vi "HFRR ADV v10.vi"() -> ()   [LabVIEW 2025] (continued)
            n3141 = local read "S 38"() -> (w4253:string)
            n3142 = local read "Temperature before test 2"() -> (w4284:dbl)
            n3143 = local read "Temperature after test 2"() -> (w4274:dbl)
            n3144 = local read "Humidity before test 2"() -> (w4299:dbl)
            n3145 = local read "Humidity after test 2"() -> (w4283:dbl)
            n3146 = local read "MWSD 2"() -> (w4288:dbl)
            n3147 = local read "WS1.4 2"() -> (w4266:dbl)
            n3148 = Concatenate Strings("2)" ("string"), w4248) -> (w4249:string)
            n3149 = Concatenate Strings("3)" ("string"), w4246) -> (w4247:string)
            n3150 = Concatenate Strings("1)" ("string"), w4253) -> (w4252:string)
            n3151 = Concatenate Strings("4)" ("string"), w4243) -> (w4244:string)
            n3152 = Concatenate Strings("5)" ("string"), w4241) -> (w4240:string)
            n3153 = Concatenate Strings("6)" ("string"), w4238) -> (w4237:string)
            n3154 = Concatenate Strings("7)" ("string"), w4234) -> (w4235:string)
            n3155 = Concatenate Strings("8)" ("string"), w4231) -> (w4232:string)
            n3156 = local read "HCF 2"() -> (w4270:dbl)
            n3157 = local read "AVP 2"() -> (w4287:dbl)
            n3158 = local read "s.NO"() -> (w4229:string)
            n3159 = call <vilib>:"New Report.vi"("report type"=enum16{"Standard Report", "HTML"}."Standard Report") -> ("report out"=w4308:refnum<class "NI_report.lvclass">, "error out"=w4307:errorcluster)  [unwired: 13 in]
            n3160 = local read "TITTLE"() -> (w4260:string)
            n3161 = Concatenate Strings(w4285, w4228, w4229, w4285, w4263, w4258, w4285, w4262, w4259, w4285, w4264, w4261, w4285) -> (w4278:string)
            "test by" <- w4278
            n3162 = Number To Fractional String(number=w4284, width (-)=i16 6, precision (6)=i16 2) -> (F-format string=w4273:string)  [unwired: 1 in]
            n3163 = Number To Fractional String(number=w4283, width (-)=i16 6, precision (6)=i16 2) -> (F-format string=w4286:string)  [unwired: 1 in]
            n3164 = Number To Fractional String(number=w4299, width (-)=i16 6, precision (6)=i16 2) -> (F-format string=w4304:string)  [unwired: 1 in]
            n3165 = Number To Fractional String(number=w4288, width (-)=i16 6, precision (6)=i16 2) -> (F-format string=w4290:string)  [unwired: 1 in]
            n3166 = Number To Fractional String(number=w4274, width (-)=i16 6, precision (6)=i16 2) -> (F-format string=w4275:string)  [unwired: 1 in]
            n3167 = Number To Fractional String(number=w4287, width (-)=i16 6, precision (6)=i16 2) -> (F-format string=w4289:string)  [unwired: 1 in]
            n3168 = Number To Fractional String(number=w4270, width (-)=i16 6, precision (6)=i16 2) -> (F-format string=w4269:string)  [unwired: 1 in]
            n3169 = Number To Fractional String(number=w4266, precision (6)=i16 2) -> (F-format string=w4265:string)  [unwired: 2 in]
            n3170 = call-dynamic "Set Report Header Text.vi"("report in"=w4308, "center header text"=w4260, "error in (no error)"=w4307) -> ("report out"=w4279:refnum<class "NI_report.lvclass">, "error out"=w4280:errorcluster)  [unwired: 11 in]
            n3171 = Concatenate Strings(w4268, w4252, w4304, w4268, w4249, w4273, w4268, w4247, w4286, w4268, w4244, w4275, w4268, w4240, w4290, w4268, w4237, w4289, w4268, w4235, w4269, w4268, w4232, w4265) -> (w4256:string)
            "export 2" <- w4256
            n3172 = call-poly <vilib>:"Append Report Text.vi"("report in"=w4279, "text"=w4278, "error in (no error)"=w4280) -> ("report out"=w4282:refnum<class "NI_report.lvclass">, "error out"=w4281:errorcluster)  [unwired: 9 in, 2 out]
            n3173 = local read "test by"() -> (w4255:string)
            n3174 = local read "TITTLE"() -> (w4257:string)
            n3175 = call-poly <vilib>:"Append Report Text.vi"("report in"=w4282, "error in (no error)"=w4281) -> ("report out"=w4303:refnum<class "NI_report.lvclass">, "error out"=w4301:errorcluster)  [unwired: 10 in, 2 out]
            n3176 = Concatenate Strings(w4257, w4256, w4255) -> (→"output":string)
            n3177 = call-poly <vilib>:"Append Report Text.vi"("report in"=w4303, "text"=w4256, "error in (no error)"=w4301) -> ("report out"=w4302:refnum<class "NI_report.lvclass">, "error out"=w4300:errorcluster)  [unwired: 9 in, 2 out]
            n3178 = call-dynamic "Print Report.vi"("report in"=w4302, "printer name (default)"=w4310, "error in (no error)"=w4300) -> ("report out"=w4312:refnum<class "NI_report.lvclass">, "error out"=w4313:errorcluster)  [unwired: 11 in]
            n3179 = call-dynamic "Dispose Report.vi"("report in"=w4312, "error in (no error)"=w4313) -> ()  [unwired: 13 in, 1 out]
          }
        }
        n3180 = case shown="True" "Print 2" {
          frame False {
          }
          frame True {
            n3181 = flat-sequence {
              frame #0 {
                n3182 = local read "s.NO"() -> (→"s.NO 2":string)
                n3183 = Wait (ms)(milliseconds to wait=u32 20) -> ()  [unwired: 1 out]
                n3184 = local read "Sample ID  3"() -> (→"Sample ID  6":string)
                n3185 = local read "Sample ID  4"() -> (→"Sample ID  7":string)
                n3186 = local read "Sample ID"() -> (→"Sample ID  2":string)
                n3187 = local read "Tested by"() -> (→"Tested by 2":string)
                n3188 = local read "Test Date"() -> (→"Test Date 2":string)
                n3189 = local read "Humidity after test 3"() -> (→"Humidity after test 4":dbl)
                n3190 = local read "Ref A Test Date :"() -> (→"TITTLE 4":string)
                n3191 = local read "Temperature before test 3"() -> (w4135:dbl)
                n3192 = local read "Temperature before test 3"() -> (→"Temperature after test 5":dbl)
                n3193 = local read "Temperature after test 3"() -> (→"Temperature after test 4":dbl)
                n3194 = local read "Humidity before test 3"() -> (→"Humidity before test 4":dbl)
                n3195 = local write "Temperature before test 3"(w4135) -> ()
                n3196 = local read "image data"() -> (w4126:T14)
                n3197 = String To Path(string="C:\\LAB-IQ\\im\\Temp_resized.jpg") -> (path=w4127:path)
                "path 2" <- w4127
                n3198 = call <vilib>:"Write JPEG File.vi"("image data"=w4126, "path to JPEG file"=w4127) -> ()  [unwired: 8 in, 2 out]
                "Ref A Test Date :" <- "Ref A Test Date :"
                "Ref B Test Date :" <- "Ref B Test Date :"
                "Ref B Scar Value :" <- "Ref B Scar Value :"
                "Ref A Scar Value :" <- "Ref A Scar Value :"
              }
              frame #1 {
                (unwired) HTML_Report_Image_Alignment."MIDDLE" ("alignment (default)")
                w4163 = u16 0 items=["portrait", "landscape"] ("orientation (portrait)")
                (unwired) HTML_Report_Image_Alignment."ABSMIDDLE" ("alignment (default)")
                (unwired) "TESTED BY : "
                (unwired) "TESTED DATE :"
                (unwired) "SAMPLE ID : "
                (unwired) "SAMPLE DESIGN : "
                w4196 = "\r"
                # "add image"
                n3199 = Wait (ms)(milliseconds to wait=u32 20) -> ()  [unwired: 1 out]
                n3200 = local read "Sample ID  2"() -> (w4189:string)
                n3201 = local read "Wear Scar X"() -> (w4161:dbl)
                "Length ( microns ) 2" <- w4161
                n3202 = local read "Wear Scar Y"() -> (w4160:dbl)
                "Wear Scar Y ( microns ) :" <- w4160
                n3203 = local read "Test Date 2"() -> (w4190:string)
                n3204 = local read "Tested by 2"() -> (w4191:string)
                n3205 = local read "String 46"() -> (w4187:string)
                n3206 = local read "String 48"() -> (w4193:string)
                n3207 = local read "String 47"() -> (w4192:string)
                n3208 = local read "String 49"() -> (w4194:string)
                n3209 = local read "String 10"() -> (w4147:string)
                n3210 = local read "s.NO 2"() -> (w4188:string)
                n3211 = Add(x=w4161, y=w4160) -> (x+y=w4159:dbl)
                n3212 = call <vilib>:"New Report.vi"("report type"=enum16{"Standard Report", "HTML"}."HTML") -> ("report out"=w4167:refnum<class "NI_report.lvclass">, "error out"=w4165:errorcluster)  [unwired: 13 in]
                n3213 = Concatenate Strings(w4196, w4187, w4188, w4196, w4193, w4189, w4196, w4192, w4190, w4196, w4194, w4191, w4196) -> (→"test by 2":string)
                n3214 = Concatenate Strings("C:\\LAB-IQ\\Data\\" ("string"), w4147, ".jpg" ("string")) -> ()  [unwired: 1 out]
                n3215 = Divide(x=w4159, y=2.0) -> (x/y=→"Mean Wear ( microns) :":dbl)
                n3216 = call-dynamic "Set Report Orientation.vi"("report in"=w4167, "orientation (portrait)"=w4163, "error in (no error)"=w4165) -> ("report out"=w4166:refnum<class "NI_report.lvclass">, "error out"=w4164:errorcluster)  [unwired: 11 in]
                n3217 = for {
                  N: 5 -> [_]
                  tunnel: w4166 -> [w4217]
                  tunnel: [w4216] -> w4145
                  tunnel: w4164 -> [w4215]
                  tunnel: [w4214] -> w4144
                  n3218 = call-dynamic "Set Report Tab Width.vi"("report in"=w4217, "error in (no error)"=w4215) -> ("report out"=w4216:refnum<class "NI_report.lvclass">, "error out"=w4214:errorcluster)  [unwired: 12 in]
                }
                n3219 = local read "TITTLE"() -> (w4162:string)
                n3220 = call-dynamic "Set Report Header Text.vi"("report in"=w4145, "center header text"=w4162, "error in (no error)"=w4144) -> ("report out"=w4183:refnum<class "NI_report.lvclass">, "error out"=w4182:errorcluster)  [unwired: 11 in]
                n3221 = for {
                  N: 1 -> [_]
                  tunnel: [w4221] -> w4169
                  tunnel: [w4220] -> w4168
                  tunnel: w4183 -> [w4219]
                  tunnel: w4182 -> [w4218]
                  n3222 = call-dynamic "New Report Line.vi"("report in"=w4219, "error in (no error)"=w4218) -> ("report out"=w4221:refnum<class "NI_report.lvclass">, "error out"=w4220:errorcluster)  [unwired: 12 in]
                }
                n3223 = for {
                  N: 2 -> [_]
                  tunnel: [w4213] -> w4175
                  tunnel: [w4212] -> w4174
                  tunnel: w4169 -> [w4211]
                  tunnel: w4168 -> [w4210]
                  n3224 = call-dynamic "New Report Line.vi"("report in"=w4211, "error in (no error)"=w4210) -> ("report out"=w4213:refnum<class "NI_report.lvclass">, "error out"=w4212:errorcluster)  [unwired: 12 in]
                }
                n3225 = for {
                  N: 25 -> [_]
                  tunnel: w4175 -> [w4209]
                  tunnel: w4174 -> [w4207]
                  tunnel: [w4208] -> w4178
                  tunnel: [w4206] -> w4177
                  n3226 = call-dynamic "Set Report Tab Width.vi"("report in"=w4209, "error in (no error)"=w4207) -> ("report out"=w4208:refnum<class "NI_report.lvclass">, "error out"=w4206:errorcluster)  [unwired: 12 in]
                }
                n3227 = control-ref of="Tab Control 9"() -> (w4173:refnum<vi>)
                n3228 = call-dynamic "Append Control Image to Report.vi"("report in"=w4178, "alignment (default)"=HTML_Report_Image_Alignment."ABSMIDDLE", "ctrl reference"=w4173, "error in (no error)"=w4177) -> ("report out"=w4172:refnum<class "NI_report.lvclass">, "error out"=w4171:errorcluster)  [unwired: 8 in, 2 out]
                n3229 = for {
                  N: 3 -> [_]
                  tunnel: [w4205] -> w4156
                  tunnel: [w4204] -> w4155
                  tunnel: w4172 -> [w4203]
                  tunnel: w4171 -> [w4202]
                  n3230 = call-dynamic "New Report Line.vi"("report in"=w4203, "error in (no error)"=w4202) -> ("report out"=w4205:refnum<class "NI_report.lvclass">, "error out"=w4204:errorcluster)  [unwired: 12 in]
                }
                n3231 = for {
                  N: 100 -> [_]
                  tunnel: w4156 -> [w4201]
                  tunnel: w4155 -> [w4199]
                  tunnel: [w4200] -> w4152
                  tunnel: [w4198] -> w4150
                  n3232 = call-dynamic "Set Report Tab Width.vi"("report in"=w4201, "error in (no error)"=w4199) -> ("report out"=w4200:refnum<class "NI_report.lvclass">, "error out"=w4198:errorcluster)  [unwired: 12 in]
                }
                n3233 = String To Path(string="C:\\LAB-IQ\\im\\Temp_resized.jpg") -> (path=w4142:path)
                n3234 = call-poly <vilib>:"Append Image to Report.vi"("report in"=w4152, "path or URL of image"=w4142, "error in (no error)"=w4150) -> ("report out"=w4151:refnum<class "NI_report.lvclass">, "error out"=w4149:errorcluster)  [unwired: 9 in, 2 out]
                n3235 = call-poly <vilib>:"Open HTML Report in Browser.vi"("report in"=w4151, "error in (no error)"=w4149) -> ("report out"=w4186:refnum<class "NI_report.lvclass">, "error out"=w4185:errorcluster)  [unwired: 11 in, 1 out]
                n3236 = call-dynamic "Dispose Report.vi"("report in"=w4186, "error in (no error)"=w4185) -> ()  [unwired: 13 in, 1 out]
              }
              frame #2 {
              }
              frame #3 {
                n3237 = disable-structure shown="Disabled" {
                  frame Disabled {
                    n3238 = local read "String 10"() -> (w4226:string)
                    n3239 = Concatenate Strings("C:\\LAB-IQ-NXT\\Data\\" ("string"), w4226, ".jpg" ("string")) -> (w4224:string)
                    n3240 = String To Path(string=w4224) -> (path=w4223:path)
                    n3241 = Delete(path (use dialog)=w4223) -> ()  [unwired: 4 in, 3 out]
                  }
                  frame Enabled {
                  }
                }
                n3242 = local write "Print 2"(FALSE ("Print")) -> ()
              }
            }
          }
        }
      }
    }
    n3243 = property on="SetTemp" class="DigNum (strict)"("Disabled"=w2110) -> ()  [unwired: 2 in, 2 out]
    n3244 = Multiply(x=w2099, y=w2101) -> (x*y=w2100:dbl)
    n3245 = local read "MWSD"() -> (w2098:dbl)
    n3246 = Add(x=w2100, y=w2098) -> (x+y=→"WS1.4":dbl)
    n3247 = Wait (ms)(milliseconds to wait=u32 50) -> ()  [unwired: 1 out]
    n3248 = Wait (ms)(milliseconds to wait=u32 50) -> ()  [unwired: 1 out]
    n3249 = local read "Quit"() -> (w2097:bool)
  }
  n3250 = VISA Close(VISA resource name=w53, error in (no error)=w52) -> (error out=w50:errorcluster)
  n3251 = VISA Close(VISA resource name=w34, error in (no error)=w33) -> ()  [unwired: 1 out]
  n3252 = call <vilib>:"Clear Errors.vi"("error in (no error)"=w50) -> ()  [unwired: 5 in, 2 out]
  n3253 = Or(x=w40, y=w39) -> (x .or. y?=w41:bool)
  n3254 = while {
    tunnel: [w4374] -> w46
    shift-right: [w4412] -> _
    shift-left: "" -> [w4400]
    tunnel: [w4388] -> _
    i -> [w4388]
    stop <- w4374 stop-if-true
    w4414 = ";" ("string")
    n3255 = local read "start en"() -> (w4433:bool)
    n3256 = And(x="st enable", y=w4433) -> (x .and. y?=w4434:bool)
    n3257 = local read "Elapsed time"() -> (w4396:dbl)
    n3258 = local read "ACQUIRE 3"() -> (w4377:bool)
    n3259 = case shown="True" w4434 {
      tunnel: "st enable" -> [w4498 w4499]
      tunnel: [w4498 w4499] -> w4378
      frame False {
      }
      frame True {
        n3260 = local write "start en"(FALSE ("start en")) -> ()
      }
    }
    n3261 = Wait (ms)(milliseconds to wait=u32 80) -> ()  [unwired: 1 out]
    n3262 = local read "Stroke"() -> (w4387:dbl)
    n3263 = Greater?(x=w4396, y=0.1) -> (0:w4394:bool)
    n3264 = Or(x=w4378, y=w4377) -> (x .or. y?=w4379:bool)
    n3265 = case shown="True" "ACQUIRE 2" {
      frame False {
      }
      frame True {
        n3266 = call "Elapsed Time13"() -> ("Time has Elapsed"=w4441:bool)  [unwired: 12 in, 7 out]
        n3267 = case shown="True" w4441 {
          frame False {
          }
          frame True {
            n3268 = local write "ACQUIRE 2"(FALSE ("ACQUIRE 2")) -> ()
            n3269 = local write "ACQUIRE 3"(FALSE ("ACQUIRE 2")) -> ()
          }
        }
        n3270 = local write "ACQUIRE 3"(TRUE ("ACQUIRE 2")) -> ()
      }
    }
    n3271 = case shown="True" w4379 {
      tunnel: w4387 -> [_ w4521]
      tunnel: [w4501 _] -> w4431
      tunnel: w4394 -> [_ _]
      tunnel: w4377 -> [_ w4508]
      frame False {
        w4501 = TRUE ("PID Rst")
        n3272 = local read "stop cmd"() -> (w4502:bool)
        n3273 = case shown="True" w4502 {
          frame False {
          }
          frame True {
            n3274 = local write "stop cmd"(FALSE ("stop cmd")) -> ()
          }
        }
        n3275 = local write "PID Rst"(TRUE ("PID Rst")) -> ()
        "start en" <- w4501
      }
      frame True {
        w4528 = cluster{"output high":dbl, "output low":dbl} {"output high"=600.0, "output low"=-600.0} ("output range")
        n3276 = local read "STROKE GAIN :"() -> (w4513:dbl)
        n3277 = call "Elapsed Time6"("Reset"="PID Rst", "Auto Reset"=FALSE) -> ("Time has Elapsed"=w4522:bool)  [unwired: 10 in, 7 out]
        n3278 = Multiply(x="Set Strk", y=w4513) -> (x*y=w4506:dbl)
        n3279 = case shown="False" w4522 {
          tunnel: [w4533 w4534] -> w4525
          tunnel: "Set Strk" -> [w4533 _]
          tunnel: w4521 -> [_ w4534]
          frame False {
          }
          frame True {
          }
        }
        n3280 = Multiply(x=w4506, y=1.0) -> (x*y=w4505:dbl)
        n3281 = Select(t=T9 {"Proportional Gain (Kc)"=0.0, "Integral Time (Ti, min)"=0.02, "Derivative Time (Td, min)"=0.0} ("Stroke PID Gains"), s=w4508, f="Stroke PID Gains") -> (s? t:f=w4509:T9)
        n3282 = Not(x=w4522) -> (.not. x?=w4520:bool)
        n3283 = call-poly <vilib>:"PID.vi"("reinitialize? (F)"=w4520, "output range"=w4528, "PID gains"=w4509, "process variable"=w4525, "setpoint"="Set Strk") -> ("output"=w4519:dbl)  [unwired: 5 in, 1 out]
        "Stroke PID OUT" <- w4519
        n3284 = Select(t=w4519, s=w4522, f=0.0) -> (s? t:f=w4523:dbl)
        n3285 = flat-sequence {
          tunnel: w4523 -> [_]
          frame #0 {
            n3286 = local write "PID Rst"(FALSE ("PID Rst")) -> ()
          }
        }
        n3287 = Add(x=w4505, y=w4523) -> (x+y=w4518:dbl)
        n3288 = Unbundle(w4528) -> ("output high"=w4527:dbl, "output low"=w4526:dbl)
        n3289 = To Word Integer(number=w4518) -> (16bit integer=w4515:i16)
        n3290 = property on="Stroke PID OUT" class="Slide (strict)"("Scale.Range:Minimum"=w4526, "Scale.Range:Maximum"=w4527) -> ()  [unwired: 2 in, 2 out]
        n3291 = In Range and Coerce(upper limit=4095.0 ("f"), x=w4515, lower limit=100.0 ("f")) -> (coerced(x)=w4512:dbl)  [unwired: 1 out]
        "PID Out" <- w4512
        n3292 = Number To Decimal String(number=w4512) -> (decimal integer string=→"st gain":string)  [unwired: 1 in]
        "stop cmd" <- TRUE ("Auto Reset")
      }
    }
    n3293 = flat-sequence {
      frame #0 {
        n3294 = local read "CH-POWER +"() -> (w4445:u16)
        n3295 = local read "CH-POWER -"() -> (w4446:u16)
        n3296 = case shown="1" w4446 {
          tunnel: "PWR" -> [w4447 w4448 w4449 w4450 w4451 w4452 w4453 w4454]
          frame 0, Default {
            n3297 = local write "Do 0"(w4447) -> ()
          }
          frame 1 {
            n3298 = local write "Do 1"(w4448) -> ()
          }
          frame 2 {
            n3299 = local write "Do 2"(w4449) -> ()
          }
          frame 3 {
            n3300 = local write "Do 3"(w4450) -> ()
          }
          frame 4 {
            n3301 = local write "Do 4"(w4451) -> ()
          }
          frame 5 {
            n3302 = local write "Do 5"(w4452) -> ()
          }
          frame 6 {
            n3303 = local write "Do 6"(w4453) -> ()
          }
          frame 7 {
            n3304 = local write "Do 7"(w4454) -> ()
          }
        }
        n3305 = case shown="1" w4445 {
          tunnel: "PWR" -> [w4455 w4456 w4457 w4458 w4459 w4460 w4461 w4462]
          frame 0, Default {
            n3306 = local write "Do 0"(w4455) -> ()
          }
          frame 1 {
            n3307 = local write "Do 1"(w4456) -> ()
          }
          frame 2 {
            n3308 = local write "Do 2"(w4457) -> ()
          }
          frame 3 {
            n3309 = local write "Do 3"(w4458) -> ()
          }
          frame 4 {
            n3310 = local write "Do 4"(w4459) -> ()
          }
          frame 5 {
            n3311 = local write "Do 5"(w4460) -> ()
          }
          frame 6 {
            n3312 = local write "Do 6"(w4461) -> ()
          }
          frame 7 {
            n3313 = local write "Do 7"(w4462) -> ()
          }
        }
      }
    }
    n3314 = local read "RUN"() -> (w4385:bool)
    n3315 = Or(x=w4385, y="ACQUIRE 3") -> (x .or. y?=w4384:bool)
    n3316 = local read "Set Hz"() -> (w4402:dbl)
    n3317 = Select(t=w4402, s=w4384, f=0.0) -> (s? t:f=w4401:dbl)
    n3318 = local read "st gain"() -> (w4405:string)
    n3319 = local read "DO"() -> (w4406:string)
    n3320 = case shown="True" "Boolean 10" {
      frame False {
      }
      frame True {
        n3321 = local write "Tab Control 8"(enum32{"setup", "calibrate"}."calibrate" ("Tab Control 8")) -> ()
        n3322 = local write "Boolean 10"(FALSE ("Boolean 10")) -> ()
      }
    }
    n3323 = Number To Decimal String(number=w4401) -> (decimal integer string=w4404:string)  [unwired: 1 in]
    n3324 = case shown="True" "Boolean 11" {
      frame False {
      }
      frame True {
        n3325 = local write "Tab Control 8"(enum32{"setup", "calibrate"}."setup" ("Tab Control 8")) -> ()
        n3326 = local write "Boolean 11"(FALSE ("Boolean 11")) -> ()
      }
    }
    n3327 = String Length(string=w4405) -> (length=w4420:i32)
    n3328 = String Length(string=w4406) -> (length=w4408:i32)
    n3329 = String Length(string=w4404) -> (length=w4421:i32)
    n3330 = Subtract(x=4.0, y=w4420) -> (x-y=w4417:dbl)
    n3331 = Subtract(x=3.0, y=w4408) -> (x-y=w4411:dbl)
    n3332 = flat-sequence {
      tunnel: w4431 -> [_]
      frame #0 {
        n3333 = Build Array("Do 0", "Do 1", "Do 2", "Do 3", "Do 4", "Do 5", "Do 6", "Do 7") -> (w4489:bool[])
        n3334 = Boolean Array To Number(Boolean array=w4489) -> (number=w4487:u32)
        n3335 = Add(x=w4487, y=u32 0) -> (x+y=w4485:u32)
        n3336 = Number To Decimal String(number=w4485) -> (decimal integer string=→"DO":string)  [unwired: 1 in]
      }
    }
    n3337 = Subtract(x=3.0, y=w4421) -> (x-y=w4422:dbl)
    n3338 = Replace Substring(3:w4417, 4:w4405, 5:"0000" ("string")) -> (1:w4415:string)  [unwired: 1 in, 1 out]
    n3339 = Replace Substring(3:w4411, 4:w4406, 5:"000" ("string")) -> (1:w4407:string)  [unwired: 1 in, 1 out]
    n3340 = Replace Substring(3:w4422, 4:w4404, 5:"000" ("string")) -> (1:w4416:string)  [unwired: 1 in, 1 out]
    n3341 = Concatenate Strings("*" ("string"), w4416, w4414, w4415, w4414, w4407, "$" ("string")) -> (w4412:string)
    "Stroke_send_Val" <- w4412
    n3342 = local read "RUN"() -> (w4382:bool)
    n3343 = local read "ACQUIRE 3"() -> (w4381:bool)
    n3344 = local read "send"() -> (w4398:bool)
    n3345 = Not Equal?(x=w4400, y=w4412) -> (x != y?=w4413:bool)
    n3346 = Or(x=w4382, y=w4381) -> (x .or. y?=w4380:bool)
    n3347 = And(x=w4398, y=w4380) -> (x .and. y?=w4397:bool)
    n3348 = Or(x=w4413, y=w4397) -> (x .or. y?=w4391:bool)
    n3349 = case shown="False" w4380 {
      frame False {
        "send" <- TRUE ("send")
      }
      frame True {
      }
    }
    n3350 = call "Elapsed Time4"("Time Target (s)"=0.5) -> ("Time has Elapsed"=w4389:bool)  [unwired: 11 in, 7 out]
    n3351 = local read "Din"() -> (w4430:u8[])
    n3352 = Or(x=w4389, y=w4391) -> (x .or. y?=w4390:bool)
    n3353 = local read "Quit"() -> (w4374:bool)
    n3354 = Index Array(array=w4430, index=0) -> (element=w4428:u8)
    n3355 = case shown="True" w4390 {
      tunnel: w4412 -> [_ w4466]
      frame False {
      }
      frame True {
        n3356 = local read "Due Com"() -> (w4467:string[])
        n3357 = Build Array (concatenate)(w4467, w4466) -> (→"Due Com":string[])
        n3358 = local write "send"(FALSE ("send")) -> ()
      }
    }
    n3359 = Number To Boolean Array(number=w4428) -> (Boolean array=w4427:bool[])
    n3360 = Array Size(array=w4427) -> (size(s)=w4426:i32)
    n3361 = Greater Than 0?(x=w4426) -> (x > 0?=w4425:bool)
    n3362 = case shown="True" w4425 {
      tunnel: w4427 -> [_ w4481]
      frame False {
      }
      frame True {
        n3363 = Index Array(array=w4481, index #1=0 ("index"), index #2=1 ("index"), index #3=2 ("index"), index #4=3 ("index"), index #5=4 ("index"), index #6=5 ("index"), index #7=6 ("index"), index #8=7 ("index")) -> (element #1=→"DI 0":bool, element #2=→"DI 1":bool, element #3=→"DI 2":bool, element #4=→"DI 3":bool, element #5=→"DI 4":bool, element #6=→"DI 5":bool, element #7=→"DI 6":bool, element #8=→"DI 7":bool)
      }
    }
  }
  n3364 = Or(x=w36, y=w41) -> (x .or. y?=w48:bool)
  n3365 = control-ref of="new picture"() -> ()  [unwired: 1 out]
  n3366 = Or(x=w55, y=w48) -> (x .or. y?=w45:bool)
  n3367 = Or(x=w45, y=w46) -> (x .or. y?=w37:bool)
  n3368 = while {
    tunnel: [w4536] -> w59
    tunnel: [w4537] -> _
    i -> [w4537]
    stop <- w4536 stop-if-true
    n3369 = local read "PID-out"() -> (w4538:dbl)
    "Horizontal Slider Control" <- w4538
    n3370 = Greater Or Equal?(x=w4538, y=2.0) -> (x >= y?=w4539:bool)
    n3371 = flat-sequence {
      tunnel: w4539 -> [w4547]
      tunnel: w4538 -> [w4550]
      tunnel: [w4548] -> w4545
      tunnel: [w4546] -> w4544
      tunnel: [w4566] -> w4543
      tunnel: w4545 -> [w4566]
      tunnel: w4544 -> [w4563]
      tunnel: [w4563] -> w4542
      tunnel: w4543 -> [w4568]
      tunnel: [w4567] -> w4541
      tunnel: w4542 -> [w4567]
      tunnel: w4541 -> [w4582]
      frame #0 {
        n3372 = case shown="True" w4547 {
          selector: w4547 -> [w4552 _]
          frame False {
            n3373 = local write "HEATER"(w4552) -> ()
          }
          frame True {
            w4554 = TRUE ("data")
            n3374 = local read "CH-HEATER"() -> (w4553:u16)
            n3375 = case shown="2" w4553 {
              tunnel: w4554 -> [w4555 w4556 w4557 w4558 w4559 w4560 w4561 w4562]
              frame 0, Default {
                n3376 = local write "Do 0"(w4555) -> ()
              }
              frame 1 {
                n3377 = local write "Do 1"(w4556) -> ()
              }
              frame 2 {
                n3378 = local write "Do 2"(w4557) -> ()
              }
              frame 3 {
                n3379 = local write "Do 3"(w4558) -> ()
              }
              frame 4 {
                n3380 = local write "Do 4"(w4559) -> ()
              }
              frame 5 {
                n3381 = local write "Do 5"(w4560) -> ()
              }
              frame 6 {
                n3382 = local write "Do 6"(w4561) -> ()
              }
              frame 7 {
                n3383 = local write "Do 7"(w4562) -> ()
              }
            }
            "HEATER" <- w4554
          }
        }
        n3384 = Select(t=w4550, s=w4547, f=0.0) -> (s? t:f=w4546:dbl)
        n3385 = Greater Or Equal?(x=w4550, y=97.0) -> (x >= y?=w4548:bool)
      }
      frame #1 {
        n3386 = Multiply(x=w4563, y=5.0) -> (x*y=w4565:dbl)
        n3387 = Wait (ms)(milliseconds to wait=w4565) -> ()  [unwired: 1 out]
      }
      frame #2 {
        n3388 = case shown="False" w4568 {
          frame False {
            w4569 = FALSE ("data")
            n3389 = local read "CH-HEATER"() -> (w4570:u16)
            n3390 = case shown="4" w4570 {
              tunnel: w4569 -> [w4571 w4572 w4573 w4574 w4575 w4576 w4577 w4578]
              frame 0, Default {
                n3391 = local write "Do 0"(w4571) -> ()
              }
              frame 1 {
                n3392 = local write "Do 1"(w4572) -> ()
              }
              frame 2 {
                n3393 = local write "Do 2"(w4573) -> ()
              }
              frame 3 {
                n3394 = local write "Do 3"(w4574) -> ()
              }
              frame 4 {
                n3395 = local write "Do 4"(w4575) -> ()
              }
              frame 5 {
                n3396 = local write "Do 5"(w4576) -> ()
              }
              frame 6 {
                n3397 = local write "Do 6"(w4577) -> ()
              }
              frame 7 {
                n3398 = local write "Do 7"(w4578) -> ()
              }
            }
            n3399 = local write "HEATER"(w4569) -> ()
          }
          frame True {
          }
        }
      }
      frame #3 {
        n3400 = Subtract(x=100, y=w4582) -> (x-y=w4581:dbl)
        n3401 = Multiply(x=w4581, y=5.0) -> (x*y=w4579:dbl)
        n3402 = Wait (ms)(milliseconds to wait=w4579) -> ()  [unwired: 1 out]
      }
    }
    n3403 = local read "Quit"() -> (w4536:bool)
  }
  n3404 = Or(x=w59, y=w37) -> (x .or. y?=w58:bool)
  n3405 = while {
    tunnel: [w4584] -> w54
    i -> [w4591]
    stop <- w4584 stop-if-true
    n3406 = local read "Quit"() -> (w4584:bool)
    n3407 = Equal To 0?(x=w4591) -> (x = 0?=w4589:bool)
    n3408 = call "Elapsed Time3"("Time Target (s)"=45.0, "Auto Reset"=TRUE) -> ("Time has Elapsed"=w4588:bool)  [unwired: 10 in, 7 out]
    n3409 = Wait (ms)(milliseconds to wait=u32 50) -> ()  [unwired: 1 out]
    n3410 = Or(x=w4588, y=w4589) -> (x .or. y?=w4590:bool)
    n3411 = case shown="True" w4590 {
      frame False {
      }
      frame True {
        n3412 = call <vilib>:"System Exec.vi"("run minimized? (F)"=TRUE, "error in (no error)"="error in (no error)", "command line"="powercfg.exe -change -monitor-timeout-ac 0") -> ("error out"=w4602:errorcluster)  [unwired: 5 in, 3 out]
        n3413 = call <vilib>:"System Exec.vi"("run minimized? (F)"=TRUE, "error in (no error)"=w4602, "command line"="powercfg.exe -change -disk-timeout-ac 0") -> ("error out"=w4601:errorcluster)  [unwired: 5 in, 3 out]
        n3414 = call <vilib>:"System Exec.vi"("run minimized? (F)"=TRUE, "error in (no error)"=w4601, "command line"="powercfg.exe -change -standby-timeout-ac 0") -> ("error out"=w4600:errorcluster)  [unwired: 5 in, 3 out]
        n3415 = call <vilib>:"System Exec.vi"("run minimized? (F)"=TRUE, "error in (no error)"=w4600, "command line"="powercfg.exe -change -hibernate-timeout-ac 0") -> ("error out"=w4599:errorcluster)  [unwired: 5 in, 3 out]
        n3416 = call <vilib>:"Simple Error Handler.vi"("error in (no error)"=w4599) -> ("error out"=w4605:errorcluster)  [unwired: 4 in, 4 out]
        n3417 = call <vilib>:"Clear Errors.vi"("error in (no error)"=w4605) -> ("error out"=→"error out":errorcluster)  [unwired: 5 in, 1 out]
      }
    }
  }
  n3418 = Compound Arithmetic op=OR(w57, w58, w54) -> (w56:bool)
  n3419 = flat-sequence {
    tunnel: w56 -> [_]
    tunnel: [w4607] -> w14
    tunnel: w14 -> [_]
    frame #0 {
      n3420 = call "CLOSE CONNECTION.vi"() -> ("error out"=w4607:errorcluster)  [unwired: 11 in]
    }
    frame #1 {
      n3421 = Quit LabVIEW(quit? (T)=TRUE) -> ()
      n3422 = local write "Quit"(FALSE ("EXIT")) -> ()
    }
  }
  n3423 = property on="Heater Button" class="Bool (strict)"("Visible"=TRUE) -> ()  [unwired: 2 in, 2 out]
  n3424 = disable-structure shown="Disabled" {
    disable-tunnel: _ -> [w4613 _]
    disable-tunnel: _ -> [w4610 _]
    disable-tunnel: _ -> [w4611 _]
    frame Disabled {
      n3425 = disable-structure shown="Disabled" {
        disable-tunnel: [w4620 _] -> w4612
        frame Disabled {
          n3426 = while {
            shift-right: [w4662] -> w4618
            shift-left: errorcluster {"status"=TRUE, "code"=0, "source"="Init"} ("error out") -> [w4627]
            shift-right: [w4661] -> w4617
            shift-left: _ -> [w4628]
            shift-right: [w4660] -> _
            shift-left: "" -> [w4659]
            tunnel: [w4621] -> w4620
            shift-right: ["Set Rh"] -> _
            shift-left: 0.0 ("Set Rh") -> [w4653]
            tunnel: [w4630] -> _
            i -> [w4630]
            stop <- w4621 stop-if-true
            n3427 = flat-sequence {
              tunnel: w4627 -> [w4665]
              tunnel: [w4665] -> w4626
              frame #0 {
                n3428 = Wait (ms)(milliseconds to wait=u32 200) -> ()  [unwired: 1 out]
              }
            }
            n3429 = local read "Com Port 3"() -> (w4629:refnum<visa-resource-name>)
            n3430 = local read "Humidity Str Rec"() -> (w4631:string)
            n3431 = Not Equal?(x="Set Rh", y=w4653) -> (x != y?=w4658:bool)
            n3432 = Number To Decimal String(number="Set Rh") -> (decimal integer string=w4656:string)  [unwired: 1 in]
            n3433 = Not Equal?(x=w4629, y=w4628) -> (x != y?=w4624:bool)
            n3434 = Concatenate Strings("#setPoint00" ("string"), w4656) -> (w4657:string)
            n3435 = case shown="False" w4658 {
              tunnel: w4657 -> [_ w4677]
              frame False {
                n3436 = local read "Humidity"() -> (w4674:bool)
                n3437 = case shown="True" w4674 {
                  frame False {
                    n3438 = local write "Humidity Str Send"("stop" ("Humidity Str Send")) -> ()
                  }
                  frame True {
                    n3439 = local write "Humidity Str Send"("start" ("Humidity Str Send")) -> ()
                  }
                }
              }
              frame True {
                n3440 = local write "Humidity Str Send"(w4677) -> ()
              }
            }
            n3441 = Or(x=w4624, y="Re-Initialise") -> (x .or. y?=w4623:bool)
            n3442 = String Subset(string=w4631, offset (0)=7) -> (substring=w4646:string)  [unwired: 1 in]
            n3443 = Match Pattern(string=w4631, regular expression="?") -> (offset past match=w4649:i32)  [unwired: 1 in, 3 out]
            n3444 = Match Pattern(string=w4631, regular expression="v") -> (offset past match=w4652:i32)  [unwired: 1 in, 3 out]
            n3445 = case shown="True" w4623 {
              tunnel: w4626 -> [w4663 _]
              tunnel: [w4663 errorcluster {"status"=TRUE, "code"=0, "source"="Init"} ("error out")] -> w4625
              frame False {
              }
              frame True {
              }
            }
            n3446 = Equal?(x=w4649, y=-1) -> (x = y?=w4633:bool)
            n3447 = Match Pattern(string=w4646, regular expression="g") -> (after substring=w4647:string, offset past match=w4638:i32)  [unwired: 1 in, 2 out]
            n3448 = Match Pattern(string=w4646, regular expression="y") -> (after substring=w4645:string, offset past match=w4639:i32)  [unwired: 1 in, 2 out]
            n3449 = Greater?(x=w4639, y=w4638) -> (0:w4644:bool)
            n3450 = Greater Or Equal To 0?(x=w4639) -> (x >= 0?=w4636:bool)
            n3451 = Greater Or Equal To 0?(x=w4638) -> (x >= 0?=w4637:bool)
            n3452 = Or(x=w4636, y=w4637) -> (x .or. y?=w4635:bool)
            n3453 = Greater Or Equal To 0?(x=w4652) -> (x >= 0?=w4634:bool)
            n3454 = Select(t=w4645, s=w4644, f=w4647) -> (s? t:f=w4640:string)
            n3455 = case shown="Error" w4625 {
              selector: w4625 -> [w4690 w4736]
              tunnel: [w4688 w4729] -> w4662
              tunnel: w4628 -> [w4691 w4735]
              tunnel: [w4689 w4738] -> w4661
              tunnel: w4659 -> [w4678 w4737]
              tunnel: [w4685 w4737] -> w4660
              frame No Error {
                n3456 = call "Elapsed Time7"() -> ("Time has Elapsed"=w4684:bool)  [unwired: 12 in, 7 out]
                n3457 = Not Equal?(x="Humidity Str Send", y=w4678) -> (x != y?=w4680:bool)
                n3458 = Or(x=w4680, y=w4684) -> (x .or. y?=w4683:bool)
                n3459 = Select(t="Humidity Str Send", s=w4680, f="vals" ("regular expression")) -> (s? t:f=w4679:string)
                n3460 = Or(x=w4683, y="Send") -> (x .or. y?=w4687:bool)
                n3461 = case shown="True" w4687 {
                  tunnel: [w4694 w4699] -> w4688
                  tunnel: w4691 -> [w4693 w4707]
                  tunnel: w4690 -> [w4694 w4706]
                  tunnel: [w4693 w4700] -> w4689
                  tunnel: w4679 -> [_ w4705]
                  tunnel: [w4692 w4696] -> w4685
                  tunnel: "Humidity Str Send" -> [_ w4697]
                  tunnel: w4680 -> [_ w4698]
                  tunnel: w4678 -> [w4692 w4695]
                  frame False {
                  }
                  frame True {
                    n3462 = flat-sequence {
                      tunnel: w4707 -> [w4715]
                      tunnel: w4706 -> [w4714]
                      tunnel: w4705 -> [w4711]
                      tunnel: [w4713] -> w4704
                      tunnel: [w4712] -> w4703
                      tunnel: w4704 -> [w4718]
                      tunnel: w4703 -> [w4717]
                      tunnel: [w4718] -> w4702
                      tunnel: [w4717] -> w4701
                      tunnel: w4702 -> [w4725]
                      tunnel: w4701 -> [w4724]
                      tunnel: [w4723] -> w4700
                      tunnel: [w4722] -> w4699
                      frame #0 {
                        n3463 = local write "Ser Led"(TRUE ("Boolean 4")) -> ()
                        n3464 = Concatenate Strings(w4711, "\r") -> (w4710:string)
                        n3465 = VISA Write(VISA resource name=w4715, write buffer=w4710, error in (no error)=w4714) -> (VISA resource name out=w4713:refnum<visa-resource-name>, error out=w4712:errorcluster)  [unwired: 1 out]
                      }
                      frame #1 {
                        n3466 = Wait (ms)(milliseconds to wait="wait") -> ()  [unwired: 1 out]
                      }
                      frame #2 {
                        w4720 = FALSE ("Send")
                        n3467 = property class="Instr"(reference=w4725, error in=w4724) -> (reference out=w4726:refnum<visa-resource-name>, error out=w4727:errorcluster, "Serial Settings:Number of Bytes at Serial Port"=w4719:u32)
                        "Humidity 2" <- w4719
                        n3468 = local write "Send"(w4720) -> ()
                        n3469 = local write "Ser Led"(w4720) -> ()
                        n3470 = VISA Read(VISA resource name=w4726, byte count=w4719, error in (no error)=w4727) -> (VISA resource name out=w4723:refnum<visa-resource-name>, read buffer=→"Humidity Str Rec":string, error out=w4722:errorcluster)  [unwired: 1 out]
                      }
                    }
                    n3471 = Select(t=w4697, s=w4698, f=w4695) -> (s? t:f=w4696:string)
                  }
                }
              }
              frame Error {
                w4743 = u16 0 items=["None"=0, "XON/XOFF"=1, "RTS/CTS"=2, "DTR/DSR"=4] ("flow control")
                w4739 = u16 0 items=["None", "Odd", "Even", "Mark", "Space"] ("parity")
                w4742 = u16 10 items=["1.0"=10, "1.5"=15, "2.0"=20] ("stop bits")
                n3472 = VISA Close(VISA resource name=w4735, error in (no error)=w4736) -> (error out=w4734:errorcluster)
                n3473 = local write "humid"("" ("humid")) -> ()
                n3474 = local write "Humidity Str Rec"("" ("Humidity Str Rec")) -> ()
                n3475 = call <vilib>:"Clear Errors.vi"("error in (no error)"=w4734) -> ("error out"=w4733:errorcluster)  [unwired: 5 in, 1 out]
                n3476 = local read "Com Port 3"() -> (w4732:refnum<visa-resource-name>)
                n3477 = call-poly "VISA Configure Serial Port"("VISA resource name"=w4732, "timeout (10sec)"=u32 1000, "termination char\n(0xA = '\\n' = LF)"=u8 10 ("termination char\n(0xA = '\\n' = LF)"), "Enable Termination\nChar (T)"=FALSE ("Enable Termination Char (T)"), "baud rate (9600)"="Humidity BaudRate", "data bits (8)"=u16 8 ("data bits"), "parity (0:none)"=w4739, "error in (no error)"=w4733, "stop bits (10: 1 bit)"=w4742, "flow control (0:none)"=w4743) -> ("VISA resource name out"=w4738:refnum<visa-resource-name>, "error out"=w4729:errorcluster)  [unwired: 4 in]
              }
            }
            n3478 = Compound Arithmetic op=AND(w4634, w4633, w4635) -> (w4632:bool)
            n3479 = case shown="True" w4632 {
              tunnel: w4631 -> [_ _]
              tunnel: w4640 -> [_ w4670]
              frame False {
              }
              frame True {
                w4668 = " " ("regular expression")
                n3480 = Match Pattern(string=w4670, regular expression=" ") -> (after substring=w4672:string)  [unwired: 1 in, 3 out]
                n3481 = Match Pattern(string=w4672, regular expression=w4668) -> (before substring=→"humid":string, after substring=w4669:string)  [unwired: 1 in, 2 out]
                n3482 = Match Pattern(string=w4669, regular expression=w4668) -> (before substring=→"temp_@Rh sensor":string)  [unwired: 1 in, 3 out]
              }
            }
            n3483 = local read "Quit"() -> (w4621:bool)
          }
          n3484 = VISA Close(VISA resource name=w4617, error in (no error)=w4618) -> (error out=w4614:errorcluster)
          n3485 = call <vilib>:"Clear Errors.vi"("error in (no error)"=w4614) -> ()  [unwired: 5 in, 2 out]
        }
        frame Enabled {
        }
      }
    }
    frame Enabled {
    }
  }
  n3486 = while {
    tunnel: [w4751] -> _
    i -> [w4751]
    stop <- w4746 stop-if-true
    # "Langauage selection"
    n3487 = property on="FF Calibration g" class="WFGraph (strict)"("Plot Area:Colors:FG Color"=u32 0) -> ()  [unwired: 2 in, 2 out]
    n3488 = Equal?(x="Lan flag", y=22.0) -> ()  [unwired: 1 out]
    n3489 = disable-structure shown="Disabled" {
      frame Disabled {
        n3490 = stacked-sequence {
          frame #0 {
            n3491 = case shown="\"Russian\"" "Language Selection" {
              tunnel: [0 1] -> w4753
              frame "English", Default {
              }
              frame "Russian" {
              }
            }
            n3492 = for {
              N: 130 -> [_]
              tunnel: "Table" -> [w4762]
              tunnel: w4753 -> [w4761]
              i -> [w4760]
              n3493 = Index Array(array=w4762, index (row)=w4760, index (col)=w4761) -> (element=w4759:string)
              n3494 = case shown="4" w4760 {
                tunnel: w4759 -> [w4763 w4764 _ w4765 w4766 w4767 w4768 w4769 w4770 w4771 w4772 w4773 w4774 w4775 w4776 w4777 w4778 w4779 w4780 w4781 w4782 w4783 w4784 w4785 w4786 w4787 w4788 w4789 w4790 _ _ w4791 w4792 w4793 w4794 w4795 w4796 w4805 w4812 w4819 w4826 w4830 w4833 w4836 w4838 w4840 w4841 w4842 w4843 w4844 w4845 w4846 w4847 w4848 w4849 w4850 w4851 w4852 w4853 w4854 w4855 w4856 w4857 w4858 w4859 w4860 w4861 w4862 w4863 w4864 w4865 w4866 w4867 w4868 w4869 w4870 w4871 w4872 w4873 w4874 w4875 w4876 w4877 w4878 w4879 w4880 w4881 w4882 w4883 w4884 w4885 w4886 w4887 w4888 w4889 w4890 w4891 w4892 w4893 w4894 w4895 w4896 w4897 w4898 w4899 _ w4900 w4901 w4902 w4903 w4904 w4905 w4906 w4907 w4908 w4909 w4910 w4911 w4912 _ w4913 w4914 w4915 w4916 w4917 w4918 _]
                frame 0 {
                  n3495 = local write "S"(w4763) -> ()
                }
                frame 1 {
                  n3496 = local write "S 2"(w4764) -> ()
                }
                frame 2 {
                }
                frame 3 {
                  n3497 = local write "S 4"(w4765) -> ()
                }
                frame 4 {
                  n3498 = property on="FILE" class="Str"("Caption.Text"=w4766) -> ()  [unwired: 2 in, 2 out]
                }
                frame 5 {
                  n3499 = property on="Fuel Discription :" class="Str"("Caption.Text"=w4767) -> ()  [unwired: 2 in, 2 out]
                }
                frame 6 {
                  n3500 = property on="Remarks :" class="Str"("Caption.Text"=w4768) -> ()  [unwired: 2 in, 2 out]
                }
                frame 7 {
                  n3501 = property on="Save & Continue" class="Bool (strict)"("Boolean Text.Text"=w4769) -> ()  [unwired: 2 in, 2 out]
                }
                frame 8 {
                }
                frame 9 {
                  n3502 = property on="Set Hz" class="DigNum (strict)"("Caption.Text"=w4771) -> ()  [unwired: 2 in, 2 out]
                }
                frame 10 {
                  "String 3" <- w4772
                }
                frame 11 {
                  n3503 = property on="NORMAL LOAD" class="DigNum (strict)"("Caption.Text"=w4773) -> ()  [unwired: 2 in, 2 out]
                }
                frame 12 {
                  "String 5" <- w4774
                }
                frame 13 {
                  n3504 = property on="Set Temp" class="DigNum (strict)"("Caption.Text"=w4775) -> ()  [unwired: 2 in, 2 out]
                }
                frame 14 {
                  n3505 = local write "S 15"(w4776) -> ()
                }
                frame 15 {
                  n3506 = property on="Set Rh" class="DigNum (strict)"("Caption.Text"=w4777) -> ()  [unwired: 2 in, 2 out]
                }
                frame 16 {
                  "String 13" <- w4778
                  "String 26" <- w4778
                }
                frame 17 {
                  n3507 = local write "S 18"(w4779) -> ()
                }
                frame 18 {
                  "String 17" <- w4780
                }
                frame 19 {
                  n3508 = property on="test time" class="DigNum (strict)"("Caption.Text"=w4781) -> ()  [unwired: 2 in, 2 out]
                }
                frame 20 {
                  "String 18" <- w4782
                  "String 22" <- w4782
                }
                frame 21 {
                  n3509 = property on="Elapsed time" class="DigNum (strict)"("Caption.Text"=w4783) -> ()  [unwired: 2 in, 2 out]
                }
                frame 22 {
                  n3510 = property on="Samplingtime 2" class="DigNum (strict)"("Caption.Text"=w4784) -> ()  [unwired: 2 in, 2 out]
                }
                frame 23 {
                  "String 21" <- w4785
                }
                frame 24 {
                  n3511 = property on="Countdown" class="DigNum (strict)"("Caption.Text"=w4786) -> ()  [unwired: 2 in, 2 out]
                }
                frame 25 {
                  n3512 = property on="Countdown 2" class="DigNum (strict)"("Caption.Text"=w4787) -> ()  [unwired: 2 in, 2 out]
                }
                frame 26 {
                  n3513 = property on="Engage" class="Bool (strict)"("Boolean Text.Text"=w4788) -> ()  [unwired: 2 in, 2 out]
                }
                frame 27 {
                  n3514 = property on="Boolean  4" class="Bool (strict)"("Boolean Text.Text"=w4789) -> ()  [unwired: 2 in, 2 out]
                }
                frame 28 {
                  n3515 = property on="Test \nStatus" class="Bool (strict)"("Boolean Text.Text"=w4790) -> ()  [unwired: 2 in, 2 out]
                }
                frame 29 {
                }
                frame 30 {
                }
                frame 31 {
                  n3516 = property on="FF Calibration g" class="WFGraph (strict)"("X Scale.Name Label.Text"=w4791) -> ()  [unwired: 2 in, 2 out]
                }
                frame 32 {
                  n3517 = property on="RSTCOF" class="Bool"("Boolean Text.Text"=w4792) -> ()  [unwired: 2 in, 2 out]
                  n3518 = property on="RST FF" class="Bool"("Boolean Text.Text"=w4792) -> ()  [unwired: 2 in, 2 out]
                  n3519 = property on="RST TEMP" class="Bool"("Boolean Text.Text"=w4792) -> ()  [unwired: 2 in, 2 out]
                  n3520 = property on="RSTV1 3" class="Bool"("Boolean Text.Text"=w4792) -> ()  [unwired: 2 in, 2 out]
                  n3521 = property on="rstv2" class="Bool"("Boolean Text.Text"=w4792) -> ()  [unwired: 2 in, 2 out]
                  n3522 = property on="RSTV1 2" class="Bool"("Boolean Text.Text"=w4792) -> ()  [unwired: 2 in, 2 out]
                  n3523 = property on="RST CP" class="Bool"("Boolean Text.Text"=w4792) -> ()  [unwired: 2 in, 2 out]
                }
                frame 33 {
                  "S 61" <- w4793
                }
                frame 34 {
                  "String 23" <- w4794
                }
                frame 35 {
                  n3524 = property on="Rh Before" class="DigNum (strict)"("Caption.Text"=w4795) -> ()  [unwired: 2 in, 2 out]
                }
                frame 36 {
                  n3525 = Match Pattern(string=w4796, regular expression=",") -> (before substring=→"bs":string, after substring=→"as":string)  [unwired: 1 in, 2 out]
                  n3526 = property on="Rh After" class="DigNum (strict)"("Caption.Text"=w4796) -> ()  [unwired: 2 in, 2 out]
                }
                frame 37 {
                  n3527 = Match Pattern(string=w4805, regular expression=",") -> (before substring=w4804:string, after substring=w4803:string)  [unwired: 1 in, 2 out]
                  "bs" <- w4804
                  "as" <- w4803
                  n3528 = Concatenate Strings(w4804, w4803) -> (w4800:string)
                  n3529 = property on="Humidity before test 2" class="DigNum (strict)"("Caption.Text"=w4800) -> ()  [unwired: 2 in, 2 out]
                  n3530 = property on="Humidity before test" class="DigNum (strict)"("Caption.Text"=w4800) -> ()  [unwired: 2 in, 2 out]
                  n3531 = Concatenate Strings(w4800, "=" ("string")) -> (w4801:string)
                  n3532 = local write "S 38"(w4801) -> ()
                }
                frame 38 {
                  n3533 = Match Pattern(string=w4812, regular expression=",") -> (before substring=w4811:string, after substring=w4810:string)  [unwired: 1 in, 2 out]
                  "bs" <- w4811
                  "as" <- w4810
                  n3534 = Concatenate Strings(w4811, w4810) -> (w4807:string)
                  n3535 = property on="Humidity after test 2" class="DigNum (strict)"("Caption.Text"=w4807) -> ()  [unwired: 2 in, 2 out]
                  n3536 = Concatenate Strings(w4807, "=" ("string")) -> (w4809:string)
                  n3537 = property on="Humidity after test" class="DigNum (strict)"("Caption.Text"=w4807) -> ()  [unwired: 2 in, 2 out]
                  n3538 = local write "S 39"(w4809) -> ()
                }
                frame 39 {
                  n3539 = Match Pattern(string=w4819, regular expression=",") -> (before substring=w4818:string, after substring=w4817:string)  [unwired: 1 in, 2 out]
                  "bs" <- w4818
                  "as" <- w4817
                  n3540 = Concatenate Strings(w4818, w4817) -> (w4814:string)
                  n3541 = property on="Temperature before test 2" class="DigNum (strict)"("Caption.Text"=w4814) -> ()  [unwired: 2 in, 2 out]
                  n3542 = property on="Temperature before test" class="DigNum (strict)"("Caption.Text"=w4814) -> ()  [unwired: 2 in, 2 out]
                  n3543 = Concatenate Strings(w4814, "=" ("string")) -> (→"String 34":string)
                }
                frame 40 {
                  n3544 = Match Pattern(string=w4826, regular expression=",") -> (before substring=w4825:string, after substring=w4824:string)  [unwired: 1 in, 2 out]
                  "bs" <- w4825
                  "as" <- w4824
                  n3545 = Concatenate Strings(w4825, w4824) -> (w4821:string)
                  n3546 = property on="Temperature after test 2" class="DigNum (strict)"("Caption.Text"=w4821) -> ()  [unwired: 2 in, 2 out]
                  n3547 = Concatenate Strings(w4821, "=" ("string")) -> (→"String 35":string)
                  n3548 = property on="Temperature after test" class="DigNum (strict)"("Caption.Text"=w4821) -> ()  [unwired: 2 in, 2 out]
                }
                frame 41 {
                  n3549 = property on="AVP" class="DigNum (strict)"("Caption.Text"=w4830) -> ()  [unwired: 2 in, 2 out]
                  n3550 = property on="AVP 2" class="DigNum (strict)"("Caption.Text"=w4830) -> ()  [unwired: 2 in, 2 out]
                  n3551 = Concatenate Strings(w4830, "=" ("string")) -> (→"String 36":string)
                }
                frame 42 {
                  n3552 = property on="MWSD" class="DigNum (strict)"("Caption.Text"=w4833) -> ()  [unwired: 2 in, 2 out]
                  n3553 = property on="MWSD 2" class="DigNum (strict)"("Caption.Text"=w4833) -> ()  [unwired: 2 in, 2 out]
                  n3554 = Concatenate Strings(w4833, "=" ("string")) -> (→"String 37":string)
                }
                frame 43 {
                  n3555 = property on="HCF 2" class="DigNum (strict)"("Caption.Text"=w4836) -> ()  [unwired: 2 in, 2 out]
                  n3556 = property on="HCF" class="DigNum (strict)"("Caption.Text"=w4836) -> ()  [unwired: 2 in, 2 out]
                  n3557 = Concatenate Strings(w4836, "=" ("string")) -> (→"String 38":string)
                }
                frame 44 {
                  n3558 = Concatenate Strings(w4838, "=" ("string")) -> (→"String 39":string)
                  n3559 = property on="WS1.4 2" class="DigNum (strict)"("Caption.Text"=w4838) -> ()  [unwired: 2 in, 2 out]
                  n3560 = property on="WS1.4" class="DigNum (strict)"("Caption.Text"=w4838) -> ()  [unwired: 2 in, 2 out]
                }
                frame 45 {
                  n3561 = property on="Save Results" class="Bool (strict)"("Boolean Text.Text"=w4840) -> ()  [unwired: 2 in, 2 out]
                }
                frame 46 {
                  n3562 = local write "S 47"(w4841) -> ()
                }
                frame 47 {
                  n3563 = local write "S 48"(w4842) -> ()
                }
                frame 48 {
                  n3564 = local write "S 49"(w4843) -> ()
                }
                frame 49 {
                  n3565 = local write "S 50"(w4844) -> ()
                }
                frame 50 {
                  n3566 = local write "S 51"(w4845) -> ()
                }
                frame 51 {
                  n3567 = local write "S 52"(w4846) -> ()
                }
                frame 52 {
                  n3568 = local write "S 53"(w4847) -> ()
                }
                frame 53 {
                  n3569 = local write "S 54"(w4848) -> ()
                }
                frame 54 {
                  n3570 = local write "S 55"(w4849) -> ()
                }
                frame 55 {
                  n3571 = local write "S 56"(w4850) -> ()
                }
                frame 56 {
                  n3572 = local write "S 57"(w4851) -> ()
                }
                frame 57 {
                  n3573 = local write "S 58"(w4852) -> ()
                }
                frame 58 {
                  n3574 = local write "S 59"(w4853) -> ()
                }
                frame 59 {
                  n3575 = local write "S 60"(w4854) -> ()
                }
                frame 60 {
                  n3576 = local write "S 62"(w4855) -> ()
                }
                frame 61 {
                  n3577 = local write "S 63"(w4856) -> ()
                }
                frame 62 {
                  n3578 = local write "S 64"(w4857) -> ()
                }
                frame 63 {
                  n3579 = local write "S 65"(w4858) -> ()
                }
                frame 64 {
                  n3580 = local write "S 66"(w4859) -> ()
                }
                frame 65 {
                  n3581 = local write "S 67"(w4860) -> ()
                }
                frame 66 {
                  n3582 = local write "S 68"(w4861) -> ()
                }
                frame 67 {
                  n3583 = local write "S 69"(w4862) -> ()
                }
                frame 68 {
                  n3584 = local write "S 70"(w4863) -> ()
                }
                frame 69 {
                  n3585 = local write "S 71"(w4864) -> ()
                }
                frame 70 {
                  n3586 = local write "S 72"(w4865) -> ()
                }
                frame 71 {
                  n3587 = local write "S 73"(w4866) -> ()
                }
                frame 72 {
                  n3588 = local write "S 74"(w4867) -> ()
                }
                frame 73 {
                  n3589 = local write "S 75"(w4868) -> ()
                }
                frame 74 {
                  n3590 = local write "S 76"(w4869) -> ()
                }
                frame 75 {
                  n3591 = local write "S 77"(w4870) -> ()
                }
                frame 76 {
                  n3592 = local write "S 78"(w4871) -> ()
                }
                frame 77 {
                  n3593 = local write "S 79"(w4872) -> ()
                }
                frame 79 {
                  n3594 = property on="Sample Temperature ( °C )" class="XYGraph (strict)"("Y Scale.Name Label.Text"=w4873) -> ()  [unwired: 2 in, 2 out]
                }
                frame 80 {
                  n3595 = local write "S 81"(w4874) -> ()
                  n3596 = property on="Humidity ( %RH )" class="XYGraph (strict)"("Y Scale.Name Label.Text"=w4874) -> ()  [unwired: 2 in, 2 out]
                }
                frame 78 {
                  n3597 = property on="Air Temperature  ( °C )" class="XYGraph (strict)"("X Scale.Name Label.Text"=w4875) -> ()  [unwired: 2 in, 2 out]
                  n3598 = property on="Humidity ( %RH )" class="XYGraph (strict)"("X Scale.Name Label.Text"=w4875) -> ()  [unwired: 2 in, 2 out]
                  n3599 = property on="Sample Temperature ( °C )" class="XYGraph (strict)"("X Scale.Name Label.Text"=w4875) -> ()  [unwired: 2 in, 2 out]
                  n3600 = property on="Coefficient Of Friction" class="XYGraph (strict)"("X Scale.Name Label.Text"=w4875) -> ()  [unwired: 2 in, 2 out]
                }
                frame 81 {
                  n3601 = property on="Air Temperature  ( °C )" class="XYGraph (strict)"("Y Scale.Name Label.Text"=w4876) -> ()  [unwired: 2 in, 2 out]
                }
                frame 82 {
                  n3602 = local write "S 84"(w4877) -> ()
                }
                frame 83 {
                  n3603 = local write "S 85"(w4878) -> ()
                }
                frame 84 {
                  n3604 = local write "S 86"(w4879) -> ()
                }
                frame 85 {
                  n3605 = local write "S 87"(w4880) -> ()
                }
                frame 86 {
                  n3606 = local write "S 88"(w4881) -> ()
                }
                frame 87 {
                  n3607 = property on="FF Calibration g" class="WFGraph (strict)"("Y Scale.Name Label.Text"=w4882) -> ()  [unwired: 2 in, 2 out]
                }
                frame 88 {
                  n3608 = local write "S 90"(w4883) -> ()
                }
                frame 89 {
                  n3609 = local write "S 91"(w4884) -> ()
                }
                frame 90 {
                  n3610 = local write "S 92"(w4885) -> ()
                }
                frame 91 {
                  n3611 = local write "S 93"(w4886) -> ()
                }
                frame 92 {
                  n3612 = local write "S 94"(w4887) -> ()
                }
                frame 93 {
                  n3613 = local write "S 95"(w4888) -> ()
                }
                frame 94 {
                  n3614 = local write "S 96"(w4889) -> ()
                }
                frame 95 {
                  n3615 = local write "S 97"(w4890) -> ()
                }
                frame 96 {
                  n3616 = local write "S 98"(w4891) -> ()
                }
                frame 97 {
                  n3617 = local write "S 99"(w4892) -> ()
                }
                frame 98 {
                  n3618 = local write "S 100"(w4893) -> ()
                }
                frame 99 {
                  n3619 = local write "S 101"(w4894) -> ()
                }
                frame 100 {
                  n3620 = local write "S 102"(w4895) -> ()
                }
                frame 101 {
                  n3621 = local write "S 103"(w4896) -> ()
                }
                frame 102 {
                  n3622 = local write "S 104"(w4897) -> ()
                }
                frame 103 {
                  n3623 = local write "S 105"(w4898) -> ()
                }
                frame 104 {
                  n3624 = local write "S 106"(w4899) -> ()
                }
                frame 105 {
                }
                frame 106 {
                  n3625 = property on="OK Button 17" class="Bool (strict)"("Boolean Text.Text"=w4900) -> ()  [unwired: 2 in, 2 out]
                }
                frame 107 {
                  n3626 = property on="OK Button 16" class="Bool (strict)"("Boolean Text.Text"=w4901) -> ()  [unwired: 2 in, 2 out]
                }
                frame 108 {
                  n3627 = property on="TITTLE" class="Str"("Caption.Text"=w4902) -> ()  [unwired: 2 in, 2 out]
                }
                frame 109 {
                  "String 30" <- w4903
                }
                frame 110 {
                  n3628 = property on="Test Date" class="Str"("Caption.Text"=w4904) -> ()  [unwired: 2 in, 2 out]
                  "String 31" <- w4904
                }
                frame 111 {
                  n3629 = property on="Sample ID" class="Str"("Caption.Text"=w4905) -> ()  [unwired: 2 in, 2 out]
                  "String 32" <- w4905
                }
                frame 112 {
                  n3630 = property on="Tested by" class="Str"("Caption.Text"=w4906) -> ()  [unwired: 2 in, 2 out]
                  "String 33" <- w4906
                }
                frame 113 {
                  n3631 = property on="System Configured Printers 2" class="Arr (strict)"("Caption.Text"=w4907) -> ()  [unwired: 2 in, 2 out]
                }
                frame 114 {
                  n3632 = property on="Selected Printer" class="Str"("Caption.Text"=w4908) -> ()  [unwired: 2 in, 2 out]
                }
                frame 115 {
